vi "ReadPath.vi"   [LabVIEW 2018]
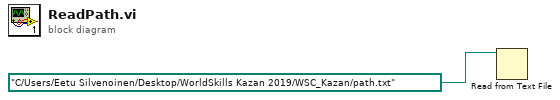
[diagram p0: block diagram]
diagram:
  n1 = Read from Text File(file (use dialog)=path "C:/Users/Eetu Silvenoinen/Desktop/WorldSkills Kazan 2019/WSC_Kazan/path.txt") -> ()  [unwired: 3 in, 4 out]
